vi "Wind_Dir_Calibration.vi"() -> ()   [LabVIEW 2012]
panel:
  out "Offset wind dir.":i32
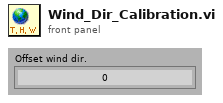
[diagram p1: front panel]
diagram:
